vi "SoundCard-Init Streaming.vi"(7 "sample rate (S/s)":dbl, 9 "Npts":i32, 11 "error in (no error)":errorcluster) -> (4 "task ID":T1 format="%.0x", 15 "error out":errorcluster)   [LabVIEW 2020]
uses:
  <vilib>/sound2/lvsound2.llb/Sound Output Task ID.ctl
  <vilib>/sound2/lvsound2.llb/Sampling Mode.ctl
  <vilib>/sound2/lvsound2.llb/Sound Data Format.ctl
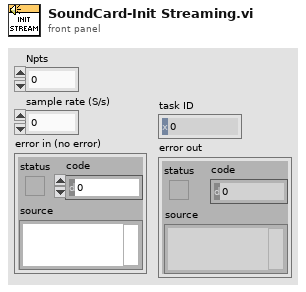
[diagram p1: front panel]
types:
  T1 = typedef "Sound Output Task ID.ctl" = u32
  T2 = typedef "Sound Data Format.ctl" = cluster{"sample rate (S/s)":dbl, "number of channels":i32, "bits per sample":i32}
  T3 = typedef "Sampling Mode.ctl" = i32
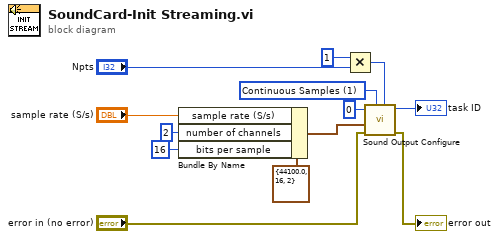
[diagram p0: block diagram]
diagram:
  w7 = T3 1 items=["Finite Samples", "Continuous Samples"] ("sample mode")
  n1 = Bundle By Name(cluster=T2 {"sample rate (S/s)"=44100.0, "number of channels"=16, "bits per sample"=2} ("sound format"), "sample rate (S/s)"="sample rate (S/s)", "number of channels"=2 ("Channels"), "bits per sample"=16) -> (w10:T2)
  n2 = Multiply(x=1, y="Npts") -> (x*y=w12:i32)
  n3 = call <vilib>:"Sound Output Configure.vi"("number of samples/ch"=w12, "sample mode"=w7, "error in (no error)"="error in (no error)", "sound format"=w10, "device ID"=u32 0) -> ("error out"=→"error out":errorcluster, "task ID"=→"task ID":T1)  [unwired: 5 in]
